vi "Table_SetDeferFrontPanelUpdates.vi"(8 "error in (no error)":errorcluster, 10 "Defer Panel Updates":bool, 11 "VI Ref":refnum<vi>) -> (0 "error out":errorcluster, 3 "VI Ref out":refnum<vi>)   [LabVIEW 2012, in "TableSupportLib.lvlib"]
uses:
  TableSupportLib.lvlib
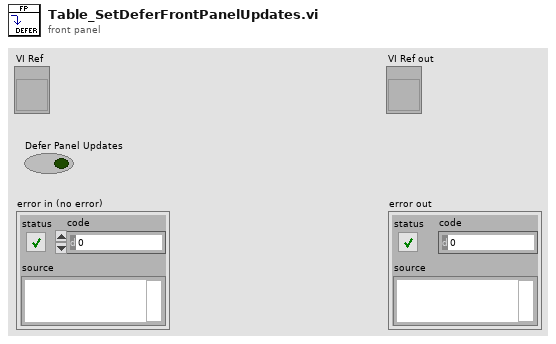
[diagram p1: front panel]
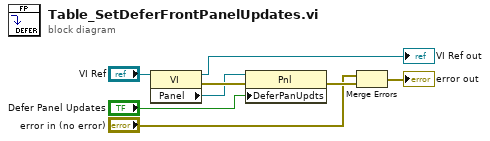
[diagram p0: block diagram]
diagram:
  n1 = property class="VI"(reference="VI Ref") -> (reference out=→"VI Ref out":refnum<vi>, error out=w5:errorcluster, "Panel"=w3:refnum<vi>)  [unwired: 1 in]
  n2 = property class="Pnl"(reference=w3, error in=w5, "DeferPanUpdts"="Defer Panel Updates") -> (error out=w7:errorcluster)  [unwired: 1 out]
  n3 = Merge Errors("error in (no error)", w7) -> (→"error out":errorcluster)
